vi "Load data.vi"(5 "File":path) -> (0 "frames":i32, 1 "Auto Data":T1(array[cluster]))   [LabVIEW 2012]
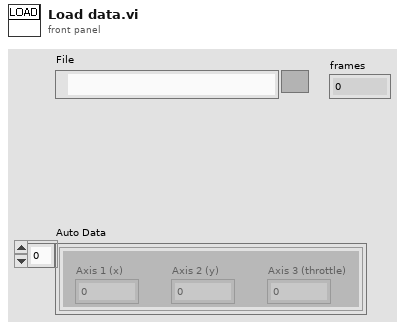
[diagram p1: front panel]
types:
  T1 = cluster{"Axis 1 (x)":dbl, "Axis 2 (y)":dbl, "Axis 3 (throttle)":dbl}[]
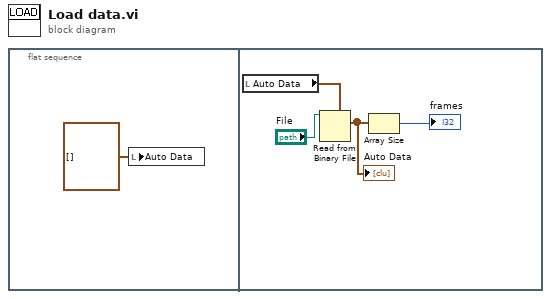
[diagram p0: block diagram]
diagram:
  n1 = flat-sequence {
    frame #0 {
      n2 = local write "Auto Data"(T1 [] ("Auto Data")) -> ()
    }
    frame #1 {
      n3 = local read "Auto Data"() -> (w3:T1)
      n4 = Read from Binary File(5:w3, 11:"File") -> (2:w2:T1)  [unwired: 4 in, 3 out]
      "Auto Data" <- w2
      n5 = Array Size(array=w2) -> (size(s)=→"frames":i32)
    }
  }
